vi "mult.vi"(0 "x":dbl, 2 "y":dbl, 5 "error in (no error)":errorcluster) -> (14 "x*y":dbl, 19 "error out":errorcluster)   [LabVIEW 2020]
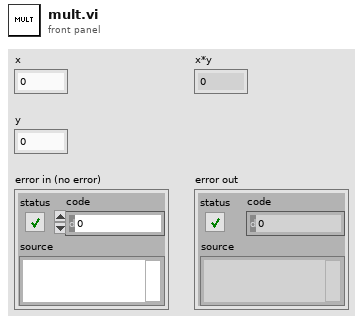
[diagram p1: front panel]
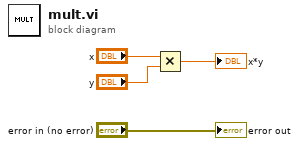
[diagram p0: block diagram]
diagram:
  n1 = Multiply(x="x", y="y") -> (x*y=→"x*y":dbl)
  "error out" <- "error in (no error)"
